vi "Teleop.vi"(10 "Match Info":T1={"Autonomous Elapsed Seconds"=0.0, "TeleOp Elapsed Seconds"=0.0, "Disabled Elapsed Seconds"=0.0, "Visited Autonomous"=FALSE, "Visited TeleOp"=FALSE, "Visited Disabled"=FALSE, "Autonomous Settings"={"Autonomous Style"=enum."Independent", "VI Refnum"=refnum}}, 11 "Call Context":T2) -> ()   [LabVIEW 2016]
doc: "This VI is called for each TeleOp packet received from the DS where the robot is not disabled. It is often used to read from the joysticks and update I/O or to update setpoints for timed control loops. It should complete and return within 20 milliseconds or it may miss DS packets."
uses:
  <vilib>/Rock Robotics/WPI/DriverStation/WPI_DriverStationDerivedRobotMode.ctl
  <vilib>/Rock Robotics/WPI/DriverStation/WPI_DriverStationMatch Info.ctl
  <vilib>/Rock Robotics/WPI/Utilities/WPI_GetSetVariantRefNum.vi
  Robot Global Data.vi
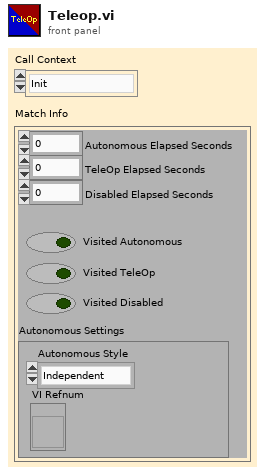
[diagram p1: front panel]
types:
  T1 = typedef "WPI_DriverStationMatch Info.ctl" = cluster{"Autonomous Elapsed Seconds":dbl, "TeleOp Elapsed Seconds":dbl, "Disabled Elapsed Seconds":dbl, "Visited Autonomous":bool, "Visited TeleOp":bool, "Visited Disabled":bool, "Autonomous Settings":cluster{"Autonomous Style":enum16{"Iterative", "Independent"}, "VI Refnum":refnum<vi>}}
  T2 = typedef "WPI_DriverStationDerivedRobotMode.ctl" = enum16{"Init", "Execute", "Stop"}
  T3 = typedef "WPI_JoystickDevRef.ctl" = cluster{"Device":T4}
  T4 = typedef "WPI_JoystickDeviceEnum.ctl" = enum16{"USB 0", "USB 1", "USB 2", "USB 3", "USB 4", "USB 5"}
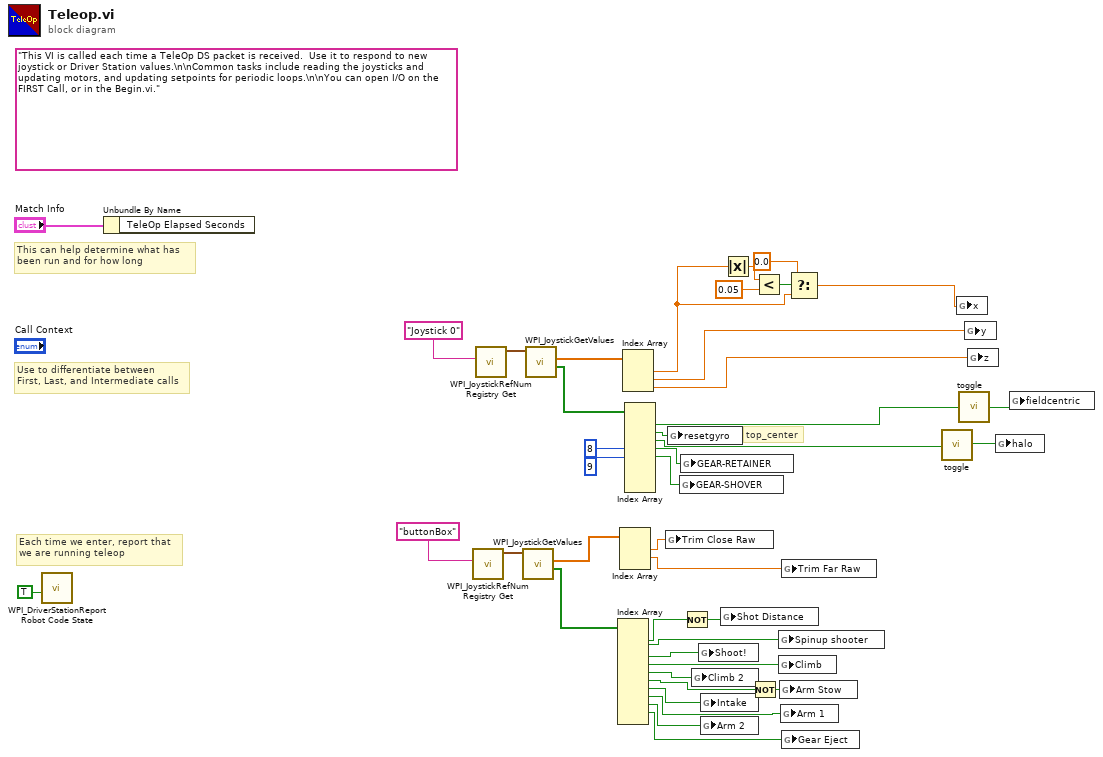
[diagram p0: block diagram]
diagram:
  (unwired) "This VI is called each time a TeleOp DS packet is received.  Use it to respond to new joystick or Driver Station values.\n\nCommon tasks include reading the joysticks and updating motors, and updating setpoints for periodic loops.\n\nYou can open I/O on the FIRST Call, or in the Begin.vi."
  # "top_center"
  # "Each time we enter, report that\nwe are running teleop"
  # "Use to differentiate between\nFirst, Last, and Intermediate calls"
  # "This can help determine what has\nbeen run and for how long"
  n1 = call <vilib>:"WPI_DriverStationReport Robot Code State.vi"("TeleOp"=TRUE ("Autonomous")) -> ()  [unwired: 10 in, 1 out]
  n2 = Unbundle By Name("Match Info") -> ()  [unwired: 1 out]
  n3 = call <vilib>:"WPI_JoystickRefNum Registry Get.vi"("refnum name"="buttonBox") -> ("JoystickDevRef"=w17:T3)  [unwired: 1 in, 9 out]
  n4 = call <vilib>:"WPI_JoystickRefNum Registry Get.vi"("refnum name"="Joystick 0") -> ("JoystickDevRef"=w39:T3)  [unwired: 1 in, 9 out]
  n5 = call <vilib>:"WPI_JoystickGetValues.vi"("JoystickDevRef"=w17) -> ("Buttons"=w15:bool[], "Axes"=w16:dbl[])  [unwired: 6 in, 3 out]
  n6 = call <vilib>:"WPI_JoystickGetValues.vi"("JoystickDevRef"=w39) -> ("Buttons"=w35:bool[], "Axes"=w37:dbl[])  [unwired: 6 in, 3 out]
  n7 = Index Array(array=w15) -> (element #1=w3:bool, element #2=w14:bool, element #3=w13:bool, element #4=w12:bool, element #5=w11:bool, element #6=w1:bool, element #7=w10:bool, element #8=w9:bool, element #9=w8:bool, element #10=w7:bool)  [unwired: 11 in, 1 out]
  n8 = Index Array(array=w16) -> (element #1=w5:dbl, element #2=w6:dbl)  [unwired: 3 in, 1 out]
  n9 = Index Array(array=w37) -> (element #1=w24:dbl, element #2=w36:dbl, element #3=w32:dbl)  [unwired: 3 in]
  n10 = Index Array(array=w35, index #4=8 ("index"), index #5=9 ("index")) -> (element #1=w29:bool, element #2=w31:bool, element #3=w30:bool, element #4=w21:bool, element #5=w20:bool)  [unwired: 7 in, 4 out]
  n11 = global write "Robot Global Data.vi" "Trim Close Raw"(w5) -> ()
  n12 = global write "Robot Global Data.vi" "resetgyro"(w31) -> ()
  n13 = global write "Robot Global Data.vi" "GEAR-SHOVER"(w20) -> ()
  n14 = global write "Robot Global Data.vi" "GEAR-RETAINER"(w21) -> ()
  n15 = Not(x=w3) -> (.not. x?=w4:bool)
  n16 = global write "Robot Global Data.vi" "Climb 2"(w11) -> ()
  n17 = global write "Robot Global Data.vi" "Shoot!"(w13) -> ()
  n18 = global write "Robot Global Data.vi" "Intake"(w10) -> ()
  n19 = global write "Robot Global Data.vi" "Arm 2"(w8) -> ()
  n20 = global write "Robot Global Data.vi" "Shot Distance"(w4) -> ()
  n21 = Absolute Value(x=w24) -> (abs(x)=w27:dbl)
  n22 = Not(x=w1) -> (.not. x?=w2:bool)
  n23 = Less?(x=w27, y=0.05) -> (x < y?=w26:bool)
  n24 = global write "Robot Global Data.vi" "Spinup shooter"(w14) -> ()
  n25 = global write "Robot Global Data.vi" "Climb"(w12) -> ()
  n26 = global write "Robot Global Data.vi" "Arm Stow"(w2) -> ()
  n27 = global write "Robot Global Data.vi" "Arm 1"(w9) -> ()
  n28 = global write "Robot Global Data.vi" "Trim Far Raw"(w6) -> ()
  n29 = global write "Robot Global Data.vi" "Gear Eject"(w7) -> ()
  n30 = Select(t=0.0, s=w26, f=w24) -> (s? t:f=w23:dbl)
  n31 = call "toggle.vi"("Input"=w30) -> ("Output"=w33:bool)
  n32 = global write "Robot Global Data.vi" "x"(w23) -> ()
  n33 = call "toggle.vi"("Input"=w29) -> ("Output"=w34:bool)
  n34 = global write "Robot Global Data.vi" "y"(w36) -> ()
  n35 = global write "Robot Global Data.vi" "z"(w32) -> ()
  n36 = global write "Robot Global Data.vi" "halo"(w33) -> ()
  n37 = global write "Robot Global Data.vi" "fieldcentric"(w34) -> ()
